vi "ActionVIOnCompile.vi"(8 "error in (no error)":errorcluster, 11 "Device Item Ref in":T1 format="%.0x") -> (0 "error out":errorcluster)   [LabVIEW 2019, in "HLA Custom Device System Explorer.lvlib"]
uses:
  HLA Custom Device System Explorer.lvlib
  <vilib>/NI VeriStand/Custom Device API/Custom Device Item Ref.ctl
  Shared/Compiled.Settings.ctl
  Shared/interaction_parameter_configuration.ctl
  Shared/object_attribute_configuration.ctl
  Shared/main_page_config.ctl
  Shared/Constants.vi
  <vilib>/NI VeriStand/Custom Device API/Get Item Property (U16).vi
  <vilib>/NI VeriStand/Custom Device API/Set Item Property (Variant).vi
  <vilib>/NI VeriStand/Custom Device API/Custom Device API.lvlib
  <vilib>/NI/NIVS Inline Async API/_Data Access System Explorer/Data Access System Explorer.lvlib
  Shared/HLA Custom Device Shared.lvlib
  <vilib>/NI VeriStand/Custom Device Tools/Custom Device Utility Library/Custom Device Utility Library.lvlib
  _Debug/VsDebugLibrary.lvlib
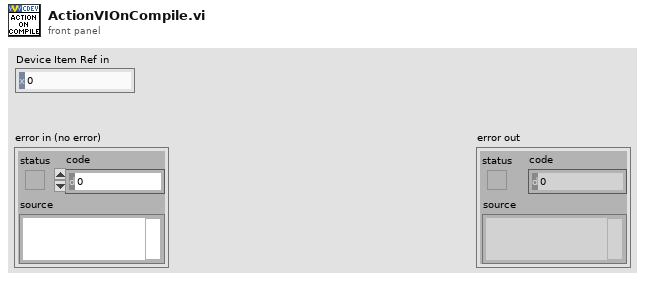
[diagram p1: front panel]
types:
  T1 = typedef "Custom Device API.lvlib/Custom Device Item Ref.ctl" = u64
  T2 = enum16{"Output/Write", "Input/Read", "Input/ReadWrite"}
  T3 = cluster{"Name":string, "Type":enum16{"Output/Write", "Input/Read", "Input/ReadWrite"}, "VS Refs":T1[]}
  T4 = typedef "HLA Custom Device Shared.lvlib/Compiled.Settings.ctl" = cluster{"Name":string, "Async Init Timeout":u16, "incoming interactions":T5[], "incoming objects":T6[], "main page properties":T7, "incoming interaction status":map{string, map{string, i32}}}
  T5 = typedef "HLA Custom Device Shared.lvlib/interaction_parameter_configuration.ctl" = cluster{"interaction name":string, "parameter name":string, "datatype":string}
  T6 = typedef "HLA Custom Device Shared.lvlib/object_attribute_configuration.ctl" = cluster{"object name":string, "instanceId":i32, "attribute name":string, "datatype":string}
  T7 = typedef "HLA Custom Device Shared.lvlib/main_page_config.ctl" = cluster{"Federate Execution Name":string, "Federate Type":string, "Local Designator Settings":string, "FOM Module":path, "mak mtl file":path}
  T8 = typedef "Custom Device API.lvlib/Custom Device File Dependency.ctl" = cluster{"Source":T9, "RT Destination":path, "ForceDownload?":bool, "SupportedTarget":T11, "Version":string}
  T9 = typedef "Custom Device API.lvlib/Path Specification.ctl" = cluster{"Path":path, "Type":T10}
  T10 = typedef "Custom Device API.lvlib/Path Type.ctl" = enum16{"Absolute", "To Base", "To Common Data Dir", "To Application Data Dir"}
  T11 = typedef "Custom Device API.lvlib/Custom Device Supported Target.ctl" = enum16{"All", "PharLap", "VxWorks", "Windows", "Linux_32_ARM", "Linux_x64", "PharLap & Windows", "PharLap & VxWorks", "VxWorks & Windows"}
  T12 = typedef "Custom Device API.lvlib/Custom Device Item Info.ctl" = cluster{"Name":string, "Is Channel":bool, "GUID":string, "Is Waveform":bool}
  T13 = cluster{"Name":string, "Type":enum16{"Output/Write", "Input/Read", "Input/ReadWrite"}, "VS Refs":T1[]}[]
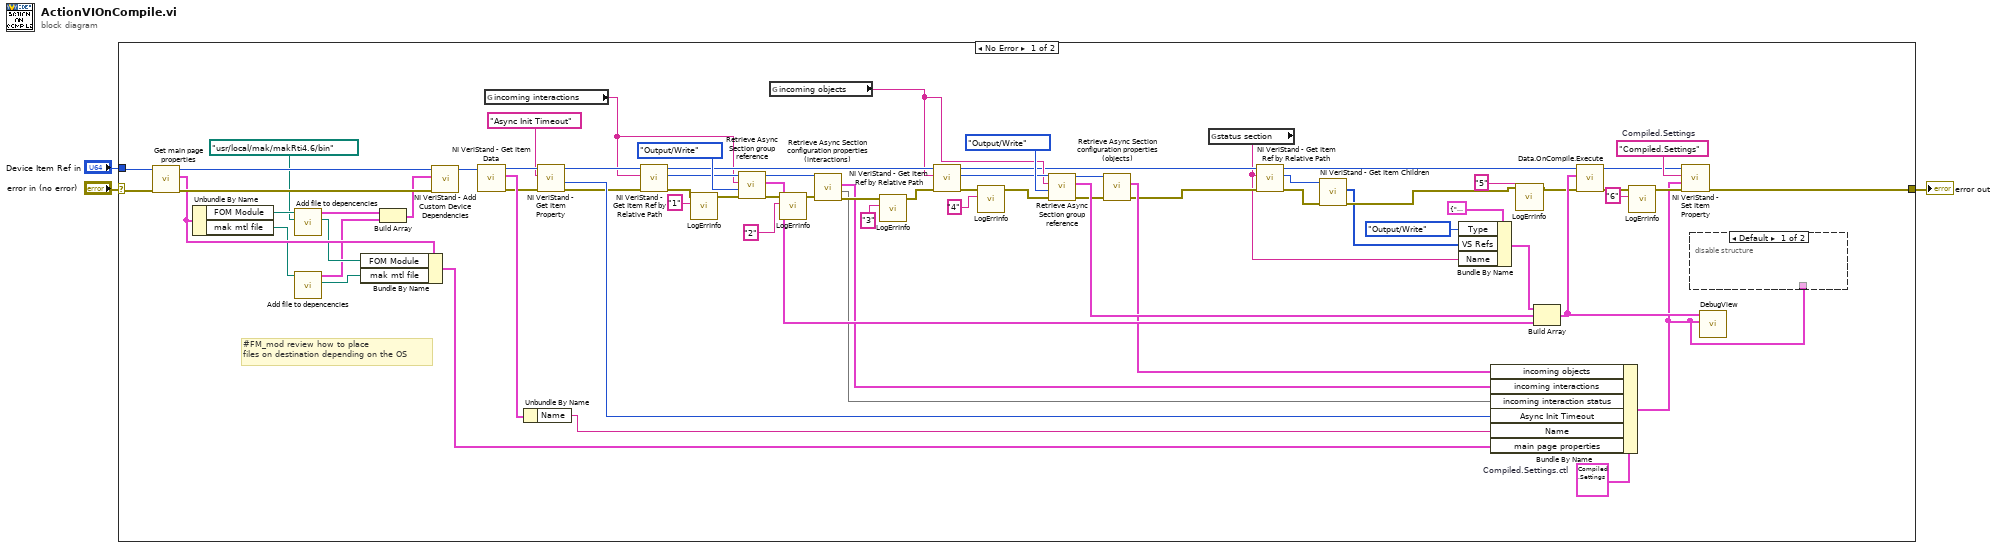
[diagram p0: block diagram]
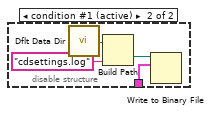
[diagram p2: hidden frame]
diagram:
  n1 = case shown="No Error" "error in (no error)" {
    selector: "error in (no error)" -> [w19 w80]
    tunnel: [w74 w80] -> w2
    tunnel: "Device Item Ref in" -> [w20 _]
    frame No Error {
      w69 = T4 {"Name"="", "Async Init Timeout"=0, "incoming interactions"=[], "incoming objects"=[], "main page properties"={"Federate Execution Name"="", "Federate Type"="", "Local Designator Settings"="", "FOM Module"=path "", "mak mtl file"=path ""}, "incoming interaction status"={}}  # Compiled.Settings.ctl
      w75 = "Compiled.Settings"  # Compiled.Settings
      # "#FM_mod review how to place\nfiles on destination depending on the OS"
      n2 = call "Get main page properties.vi"("error in"=w19, "Item Ref in"=w20) -> ("error out"=w16:errorcluster, "main page properties"=w12:T7, "Item Ref out"=w18:T1)  [unwired: 7 in]
      n3 = Unbundle By Name(w12) -> ("FOM Module"=w15:path, "mak mtl file"=w7:path)
      n4 = call "Add file to depencencies.vi"("RT Destination folder (c:\\ni-rt\\NIVeriStand)"=path "/usr/local/mak/makRti4.6/bin" ("RT Destination folder (c:\\ni-rt\\NIVeriStand)"), "item path"=w15) -> ("destination path"=w10:path, "dependency out"=w14:T8)  [unwired: 8 in]
      n5 = call "Add file to depencencies.vi"("item path"=w7) -> ("destination path"=w9:path, "dependency out"=w8:T8)  [unwired: 9 in]
      n6 = Bundle By Name(cluster=w12, "FOM Module"=w10, "mak mtl file"=w9) -> (w11:T7)
      n7 = Build Array(w14, w8) -> (w13:T8[])
      n8 = call <vilib>:"NI VeriStand - Add Custom Device Dependencies.vi"("error in (no error)"=w16, "Dependencies"=w13, "Device Ref in"=w18) -> ("Device Ref out"=w17:T1)  [unwired: 7 in, 1 out]
      n9 = call <vilib>:"NI VeriStand - Get Item Data.vi"("Item Ref in"=w17) -> ("error out"=w68:errorcluster, "Item Info"=w73:T12, "Item Ref out"=w67:T1)  [unwired: 7 in, 1 out]
      n10 = global read "Constants.vi" "incoming interactions"() -> (w49:string)
      n11 = Unbundle By Name(w73) -> ("Name"=w72:string)
      n12 = call-poly <vilib>:"NI VeriStand - Get Item Property.vi"("error in (no error)"=w68, "Property Name"="Async Init Timeout", "Item Ref in"=w67) -> ("error out"=w56:errorcluster, "Value"=w65:u16, "Item Ref out"=w57:T1)  [unwired: 5 in, 1 out]
      n13 = call <vilib>:"NI VeriStand - Get Item Ref by Relative Path.vi"("error in"=w56, "Relative Item Path"=w49, "Section Ref in"=w57) -> ("error out"=w55:errorcluster, "Item Ref"=w52:T1, "Section Ref out"=w53:T1)  [unwired: 5 in, 1 out]
      n14 = call "LogErrInfo.vi"("location info"="1", "error in (no error)"=w55) -> ("error out"=w47:errorcluster)  [unwired: 9 in]
      n15 = call "Retrieve Async Section group reference.vi"("error in"=w47, "Type"=T2."Output/Write", "async session name"=w49, "section item ref in"=w52) -> ("error out"=w59:errorcluster, "vs group ref"=w63:T3, "section item ref out"=w60:T1)  [unwired: 4 in, 1 out]
      n16 = global read "Constants.vi" "incoming objects"() -> (w48:string)
      n17 = call "LogErrInfo.vi"("location info"="2", "error in (no error)"=w59) -> ("error out"=w45:errorcluster)  [unwired: 9 in]
      n18 = call "Retrieve Async Section configuration properties (interactions).vi"("error in"=w45, "section item ref in"=w60) -> ("error out"=w54:errorcluster, "status channel configuration"=w4:map{string, map{string, i32}}, "data channel configuration"=w33:T5[])  [unwired: 5 in, 2 out]
      n19 = call "LogErrInfo.vi"("location info"="3", "error in (no error)"=w54) -> ("error out"=w44:errorcluster)  [unwired: 9 in]
      n20 = call <vilib>:"NI VeriStand - Get Item Ref by Relative Path.vi"("error in"=w44, "Relative Item Path"=w48, "Section Ref in"=w53) -> ("error out"=w50:errorcluster, "Item Ref"=w51:T1, "Section Ref out"=w31:T1)  [unwired: 5 in, 1 out]
      n21 = call "LogErrInfo.vi"("location info"="4", "error in (no error)"=w50) -> ("error out"=w43:errorcluster)  [unwired: 9 in]
      n22 = call "Retrieve Async Section group reference.vi"("error in"=w43, "Type"=T2."Output/Write", "async session name"=w48, "section item ref in"=w51) -> ("error out"=w35:errorcluster, "vs group ref"=w61:T3, "section item ref out"=w34:T1)  [unwired: 4 in, 1 out]
      n23 = call "Retrieve Async Section configuration properties (objects).vi"("error in"=w35, "section item ref in"=w34) -> ("error out"=w28:errorcluster, "configuration properties"=w32:T6[])  [unwired: 6 in, 2 out]
      n24 = global read "Constants.vi" "status section"() -> (w21:string)
      n25 = call <vilib>:"NI VeriStand - Get Item Ref by Relative Path.vi"("error in"=w28, "Relative Item Path"=w21, "Section Ref in"=w31) -> ("error out"=w27:errorcluster, "Item Ref"=w23:T1, "Section Ref out"=w24:T1)  [unwired: 5 in, 1 out]
      n26 = call <vilib>:"NI VeriStand - Get Item Children.vi"("error in (no error)"=w27, "Item Ref in"=w23) -> ("error out"=w26:errorcluster, "Child Refs"=w22:T1[])  [unwired: 6 in, 2 out]
      n27 = Bundle By Name(cluster=T3 {"Name"="", "Type"=enum."Output/Write", "VS Refs"=[]} ("Group"), "Type"=T2."Output/Write", "VS Refs"=w22, "Name"=w21) -> (w29:T3)
      n28 = Bundle By Name(cluster=w69, "incoming objects"=w32, "incoming interactions"=w33, "incoming interaction status"=w4, "Async Init Timeout"=w65, "Name"=w72, "main page properties"=w11) -> (w5:T4)
      n29 = call "LogErrInfo.vi"("location info"="5", "error in (no error)"=w26) -> ("error out"=w42:errorcluster)  [unwired: 9 in]
      n30 = Build Array(w29, w61, w63) -> (w58:T13)
      n31 = call <vilib>:"Data.OnCompile.Execute.vi"("error in"=w42, "VS Ref Groups"=w58, "Custom Device Ref"=w24) -> ("error out"=w71:errorcluster, "Custom Device Ref"=w70:T1)  [unwired: 7 in]
      n32 = call "LogErrInfo.vi"("location info"="6", "error in (no error)"=w71) -> ("error out"=w37:errorcluster)  [unwired: 9 in]
      n33 = call-poly <vilib>:"NI VeriStand - Set Item Property.vi"("error in (no error)"=w37, "Value"=w5, "Property Name"=w75, "Item Ref in"=w70) -> ("error out"=w74:errorcluster)  [unwired: 5 in, 2 out]
      n34 = disable-structure shown="Default" {
        disable-tunnel: w5 -> [_ w76]
        frame condition #0 {
        }
        frame condition #1 (active) {
          n35 = call <vilib>:"Dflt Data Dir.vi"() -> ("App:Default Data Directory"=w79:path)
          n36 = Build Path(base path=w79, name or relative path="cdsettings.log") -> (appended path=w78:path)
          n37 = Write to Binary File(file (use dialog)=w78, data=w76) -> ()  [unwired: 4 in, 3 out]
        }
      }
      n38 = call "DebugView.vi"("Compiled.Settings.ctl"=w5, "appended array"=w58) -> ()  [unwired: 10 in]
    }
    frame Error {
    }
  }
  "error out" <- w2
